vi "Generate ShowInterface Event.vi"(8 "error in (no error)":errorcluster, 9 "Data":variant, 10 "Event Type":T1=enum."Initialize Finish", 11 "Sender":string) -> (0 "error out":errorcluster)   [LabVIEW 2010]
uses:
  Event Type.ctl
  Interface Template Event.lvlib
panel:
  # "Input"
  # "Output"
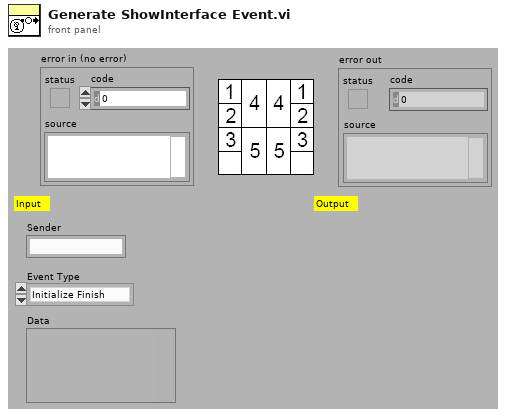
[diagram p1: front panel]
types:
  T1 = typedef "Interface Template Event.lvlib/Event Type.ctl" = enum16{"Default", "Initialize Finish", "Button 0 Click", "Exit Click", "Exit"}
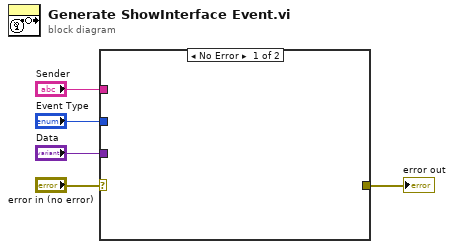
[diagram p0: block diagram]
diagram:
  n1 = case shown="No Error" "error in (no error)" {
    selector: "error in (no error)" -> [_ w6]
    tunnel: [_ w6] -> w2
    tunnel: "Event Type" -> [_ _]
    tunnel: "Data" -> [_ _]
    tunnel: "Sender" -> [_ _]
    frame No Error {
    }
    frame Error {
    }
  }
  "error out" <- w2
